vi "Emballage_BDD_Chargement_config_Flatprop.vi"(8 "Error in":errorcluster caption="Error in (no error)") -> (0 "Error out":errorcluster)   [LabVIEW 2020]
uses:
  Modules/FS/60_FS_Controles/60_FS_SetGet.ctl
panel:
  out "Chaîne_progress 2":string
  out "progress 2":u8(slide) scale=0.0..100.0
  out "Chaîne_progress":string
  out "Tableau_config_Flatprop":string[][](array[string])
  out "progress":u8(slide) scale=0.0..100.0
  out "listeXml":string[](array[string])
  out "taille(s)":i32
  out "repertoireConfigs":path
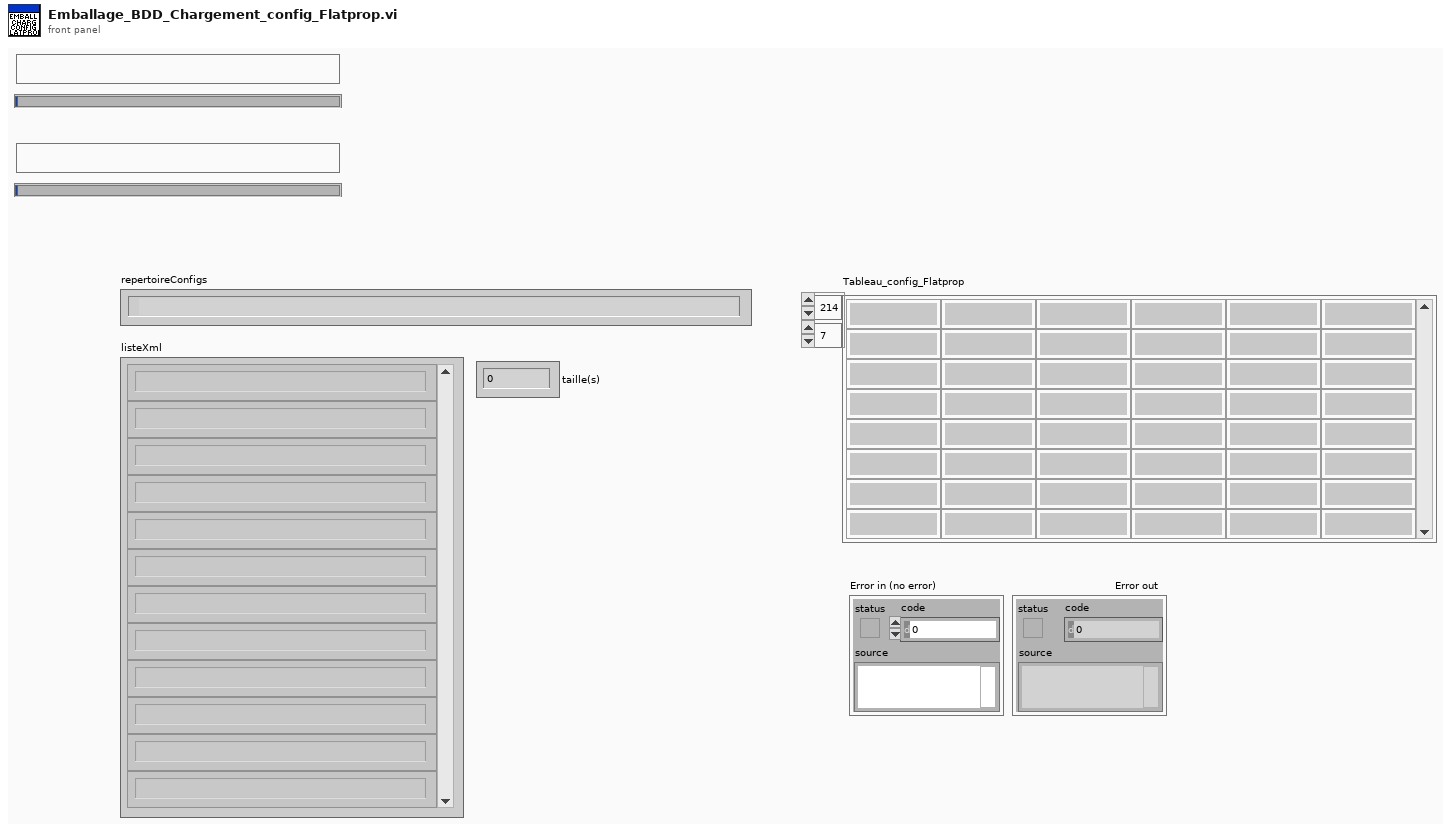
[diagram p1: front panel]
types:
  T1 = typedef "60_FS_SetGet.ctl" = enum16{"set", "get"}
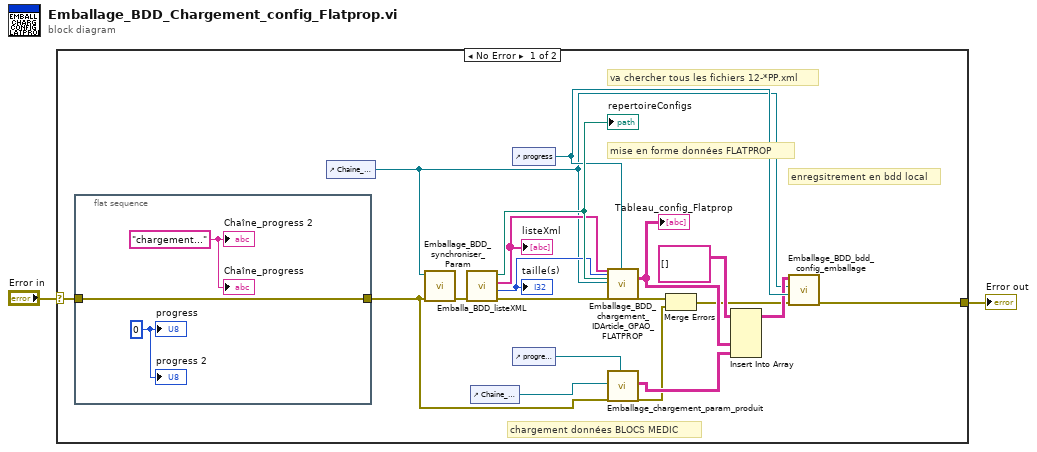
[diagram p0: block diagram]
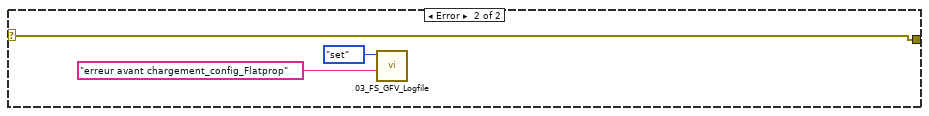
[diagram p2: hidden frame]
diagram:
  n1 = case shown="No Error" "Error in" {
    selector: "Error in" -> [w18 w27]
    tunnel: [w10 w27] -> w1
    frame No Error {
      # "chargement données BLOCS MEDIC"
      # "enregsitrement en bdd local"
      # "mise en forme données FLATPROP"
      # "va chercher tous les fichiers 12-*PP.xml"
      n2 = flat-sequence {
        tunnel: w18 -> [w24]
        tunnel: [w24] -> w8
        frame #0 {
          w22 = "chargement..." ("Chaîne_progress")
          w23 = u8 0 ("progress")
          "progress" <- w23
          "Chaîne_progress" <- w22
          "progress 2" <- w23
          "Chaîne_progress 2" <- w22
        }
      }
      n3 = control-ref of="Chaîne_progress"() -> (w11:refnum<vi>)
      n4 = call "Emballage_BDD_synchroniser_Param.vi"("error in (no error)"=w8, "Refnum Ch"=w11) -> ("error out"=w12:errorcluster)  [unwired: 9 in]
      n5 = call "Emballa_BDD_listeXML.vi"("entrée d'erreur (pas d'erreur)"=w12) -> ("sortie d'erreur"=w9:errorcluster, "Numérique"=w19:i32, "filenames"=w20:string[], "repertoireConfigs"=w21:path)  [unwired: 7 in]
      "listeXml" <- w20
      "taille(s)" <- w19
      "repertoireConfigs" <- w21
      n6 = control-ref of="Chaîne_progress 2"() -> (w4:refnum<vi>)
      n7 = control-ref of="progress"() -> (w17:refnum<vi>)
      n8 = control-ref of="progress 2"() -> (w5:refnum<vi>)
      n9 = call "Emballage_BDD_chargement_IDArticle_GPAO_FLATPROP.vi"("filenames"=w20, "taille"=w19, "repertoireConfigs"=w21, "Refnum Ch"=w11, "entrée d'erreur (pas d'erreur)"=w9, "progress"=w17) -> ("Tableau en sortie"=w16:string[][], "sortie d'erreur"=w6:errorcluster)  [unwired: 8 in, 12 out]
      "Tableau_config_Flatprop" <- w16
      n10 = call "Emballage_chargement_param_produit.vi"("Refnum Ch"=w4, "entrée d'erreur (pas d'erreur)"=w8, "progress"=w5) -> ("Tableau en sortie"=w15:string[][], "sortie d'erreur"=w3:errorcluster)  [unwired: 15 in]
      n11 = Merge Errors(w6, w3) -> (w7:errorcluster)
      n12 = Insert Into Array(array=string[][] [] ("tableau"), new element #1=w16, new element #2=w15) -> (w13:string[][])  [unwired: 2 in]
      n13 = call "Emballage_BDD_bdd_config_emballage.vi"("Error in"=w7, "progress"=w17, "Refnum Ch"=w11, "tableau_config"=w13) -> ("Error out"=w10:errorcluster)  [unwired: 6 in, 1 out]
    }
    frame Error {
      n14 = call "03_FS_GFV_Logfile.vi"("Chaîne"="erreur avant chargement_config_Flatprop", "States"=60_FS_SetGet."set") -> ()  [unwired: 8 in, 2 out]
    }
  }
  "Error out" <- w1
